vi "Delete Emitter.vi"(8 "error in (no error)":errorcluster, 10 "Emitter":string, 11 "Controller in":refnum<class "Controller.lvclass">) -> (0 "error out":errorcluster, 3 "Controller out":refnum<class "Controller.lvclass">)   [LabVIEW 2014, in "Controller.lvlib" / "Controller.lvclass"]
uses:
  Controller.lvclass
  Controller.lvclass/Controller.ctl
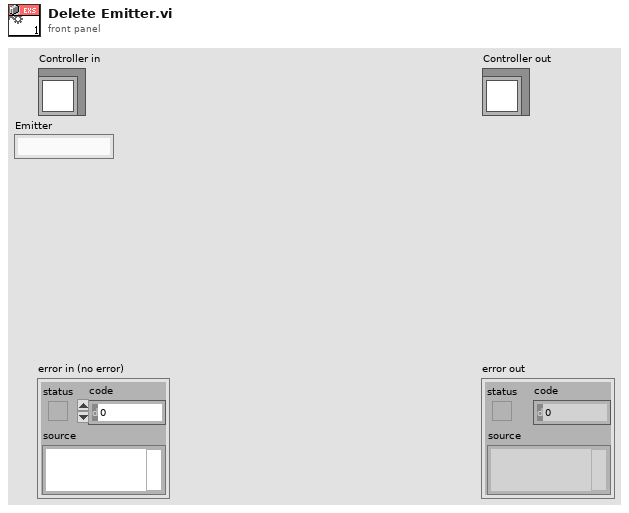
[diagram p1: front panel]
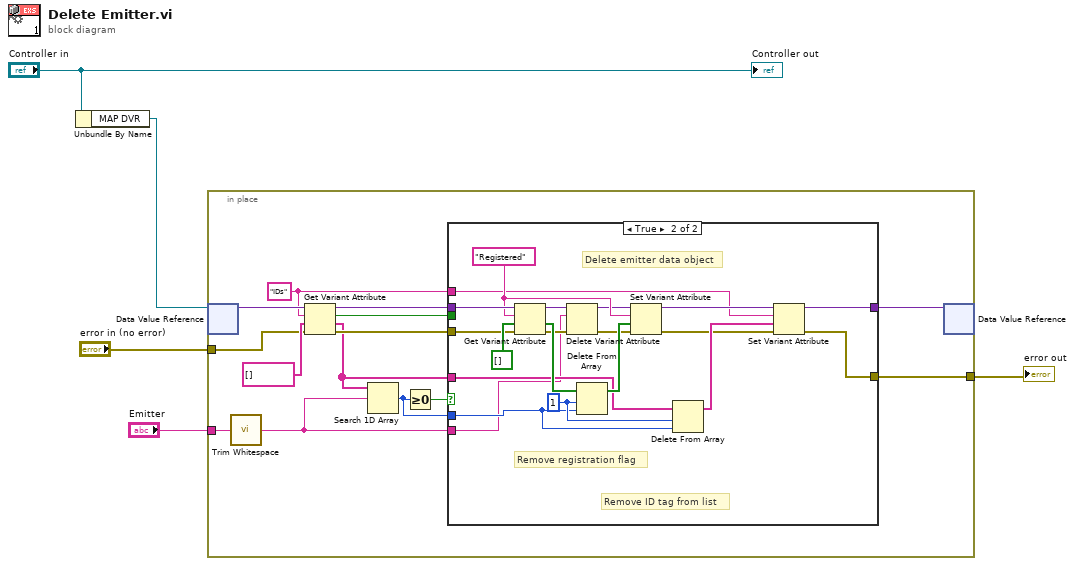
[diagram p0: block diagram]
diagram:
  n1 = Unbundle By Name("Controller in") -> ("MAP DVR"=w4:refnum<data-value>)
  n2 = in-place {
    in-place-border: "Emitter" -> [w10]
    in-place-border: "error in (no error)" -> [w13]
    in-place-border: [w11] -> w1
    w16 = "IDs" ("name")
    n3 = in-place-dvr #1(w4) -> (w19:variant)  [unwired: 1 out]
    n4 = call <vilib>:"Trim Whitespace.vi"("string"=w10) -> ("trimmed string"=w8:string)  [unwired: 1 in]
    n5 = Get Variant Attribute(Variant=w19, name=w16, default value (empty Variant)=string[] [], error in=w13) -> (duplicate Variant=w15:variant, found=w17:bool, value=w9:string[], error out=w14:errorcluster)
    n6 = Search 1D Array(1D array=w9, element=w8) -> (index of element=w6:i32)  [unwired: 1 in]
    n7 = Greater Or Equal To 0?(x=w6) -> (x >= 0?=w7:bool)
    n8 = case shown="True" w7 {
      tunnel: w17 -> [_ _]
      tunnel: w9 -> [_ w27]
      tunnel: w16 -> [_ w25]
      tunnel: w15 -> [w21 w40]
      tunnel: w14 -> [w20 w38]
      tunnel: [w21 w28] -> w12
      tunnel: [w20 w23] -> w11
      tunnel: w8 -> [_ w22]
      tunnel: w6 -> [_ w30]
      frame False {
        # "Emitters can already be registered if an actor is launched and returning data before this is run.  Prevent multiple registration..."
      }
      frame True {
        w31 = 1 ("length")
        w39 = "Registered" ("name")
        # "Delete emitter data object"
        # "Remove ID tag from list"
        # "Remove registration flag"
        n9 = Get Variant Attribute(Variant=w40, name=w39, default value (empty Variant)=bool[] [], error in=w38) -> (duplicate Variant=w35:variant, value=w37:bool[], error out=w34:errorcluster)  [unwired: 1 out]
        n10 = Delete Variant Attribute(4:w34, 6:w22, 7:w35) -> (0:w32:errorcluster, 3:w33:variant)  [unwired: 1 out]
        n11 = Delete From Array(array=w37, length=w31, index=w30) -> (array with subset deleted=w36:bool[])  [unwired: 1 out]
        n12 = Set Variant Attribute(Variant=w33, name=w39, value=w36, error in=w32) -> (Variant out=w29:variant, error out=w24:errorcluster)  [unwired: 1 out]
        n13 = Delete From Array(array=w27, length=w31, index=w30) -> (array with subset deleted=w26:string[])  [unwired: 1 out]
        n14 = Set Variant Attribute(Variant=w29, name=w25, value=w26, error in=w24) -> (Variant out=w28:variant, error out=w23:errorcluster)  [unwired: 1 out]
      }
    }
    n15 = in-place-dvr #1(w12) -> ()  [unwired: 2 out]
  }
  "error out" <- w1
  "Controller out" <- "Controller in"
